vi "main.vi"() -> ()   [LabVIEW 2011]
uses:
  Sliding Menu/Sliding Menu Library/Sliding Menu xControl/Sliding Menu XControl.xctl
  Framework SubVIs/Main Type Definitions/User Interface Type Definitions.ctl
  Framework SubVIs/Main Type Definitions/UI Picture Containers.ctl
  Framework SubVIs/User Interface/UI Control Definitions/UI Configuration Information.ctl
  Framework SubVIs/Plugin Handler/Plugin Command Manager/Plugin Initialize/Plugin Handler Initialize.lvclass
  Framework SubVIs/Plugin Handler/Plugin Command Manager/Plugin Handler Command.lvclass
  Framework SubVIs/User Interface/UI Command Manager/UI Command Manager.lvclass
  Framework SubVIs/User Interface/UI Command Manager/UI Initialize/UI Initialize.lvclass
  Framework SubVIs/Plugin Handler/Plugin Command Manager/Plugin Handler Stop/Plugin Handler Stop.lvclass
  Framework SubVIs/User Interface/UI Command Manager/UI Command Manager Stop/UI Command Manager Stop.lvclass
  Framework SubVIs/User Interface/UI Command Manager/UI Resize Menu/Resize Menu.lvclass
  Framework SubVIs/Plugin Handler/Plugin Command Manager/Plugin Display UI/Plugin Display UI.lvclass
  Framework SubVIs/User Interface/UI Command Manager/UI Toggle Menu/UI Toggle Menu.lvclass
  Framework SubVIs/Plugin Handler/Plugin Command Manager/Plugin Launch Next/Plugin Load Next.lvclass
panel:
  out "Time":string
  in  "Name":string
  out "Header Image":picture
  in  "Tab Control":enum32{"Page 1", "Page 2"}(tab)
  out "Sliding Menu XControl":i32(xcontrol)
  in  "Go Home":bool
  in  "Lock Interface":bool caption="Boolean 2"
  in  "Menu":bool
  out "Footer Image":picture
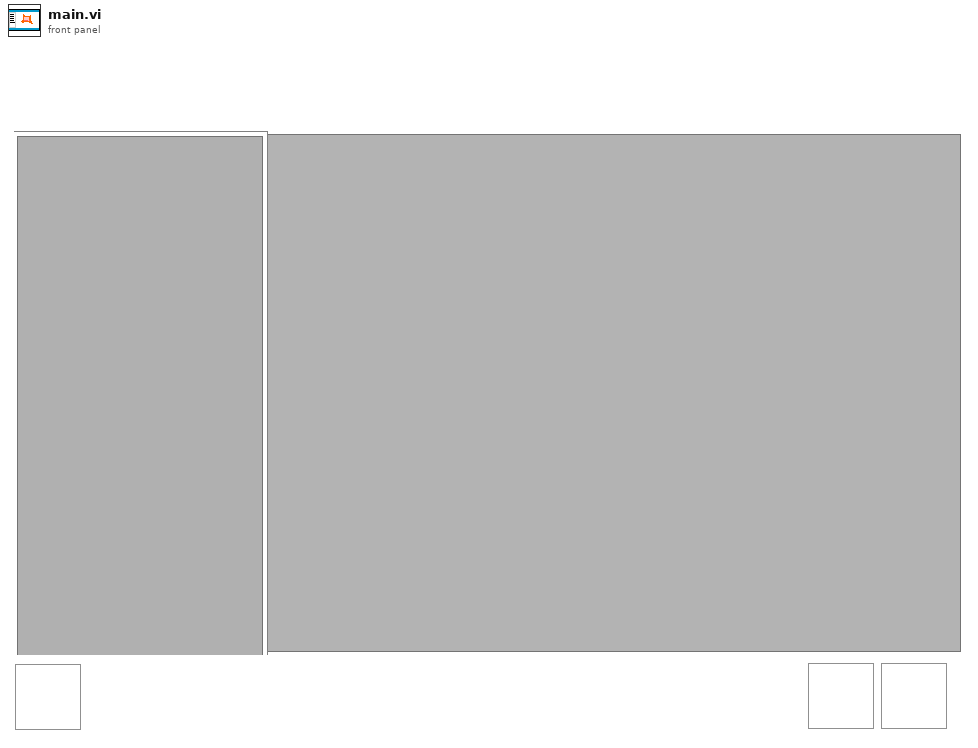
[diagram p1: front panel]
types:
  T1 = typedef "User Interface Type Definitions.ctl" = cluster{"This VI":refnum<vi>, "User Interace Plugin":refnum<vi>, "UI Picture Container References":T2, "Sliding Menu XControl":refnum<vi>, "Menu Container":refnum<vi>, "UI Configuration Information":T3, "Header Text":refnum<vi>}
  T2 = typedef "UI Picture Containers.ctl" = cluster{"Header Image":refnum<vi>, "Footer Image":refnum<vi>}
  T3 = typedef "UI Configuration Information.ctl" = cluster{"Space Between Buttons":i32, "Number of Buttons to Show":i32, "Header Image":path, "Footer Image":path}
  T4 = cluster{"Header Image":refnum<vi>, "Footer Image":refnum<vi>}
  T5 = typedef "Framework Configuration Data.ctl" = cluster{"Plugin Configuration Information":T6, "UI Configuration Information":T3}
  T6 = typedef "Plugin Configuration Information.ctl" = cluster{"Plugin Locaiton on Disk":path}
  T7 = typedef "Plugin Handler Shifter Data Definition.ctl" = cluster{"Array of Plugins":refnum<class "Generic Plugin.lvclass">[], "Plugin Configuration Information":T6, "UI Queue":refnum<queue>, "Shutdown Event":refnum<user-event>, "Menu Open Event":refnum<user-event>, "Menu Closed Event":refnum<user-event>, "Index of Plugin Showing":i32}
  T8 = enum32{"invalid app kind", "Development System", "Run Time System", "Student Edition", "Embedded LabVIEW", "Evaluation", "Custom"}
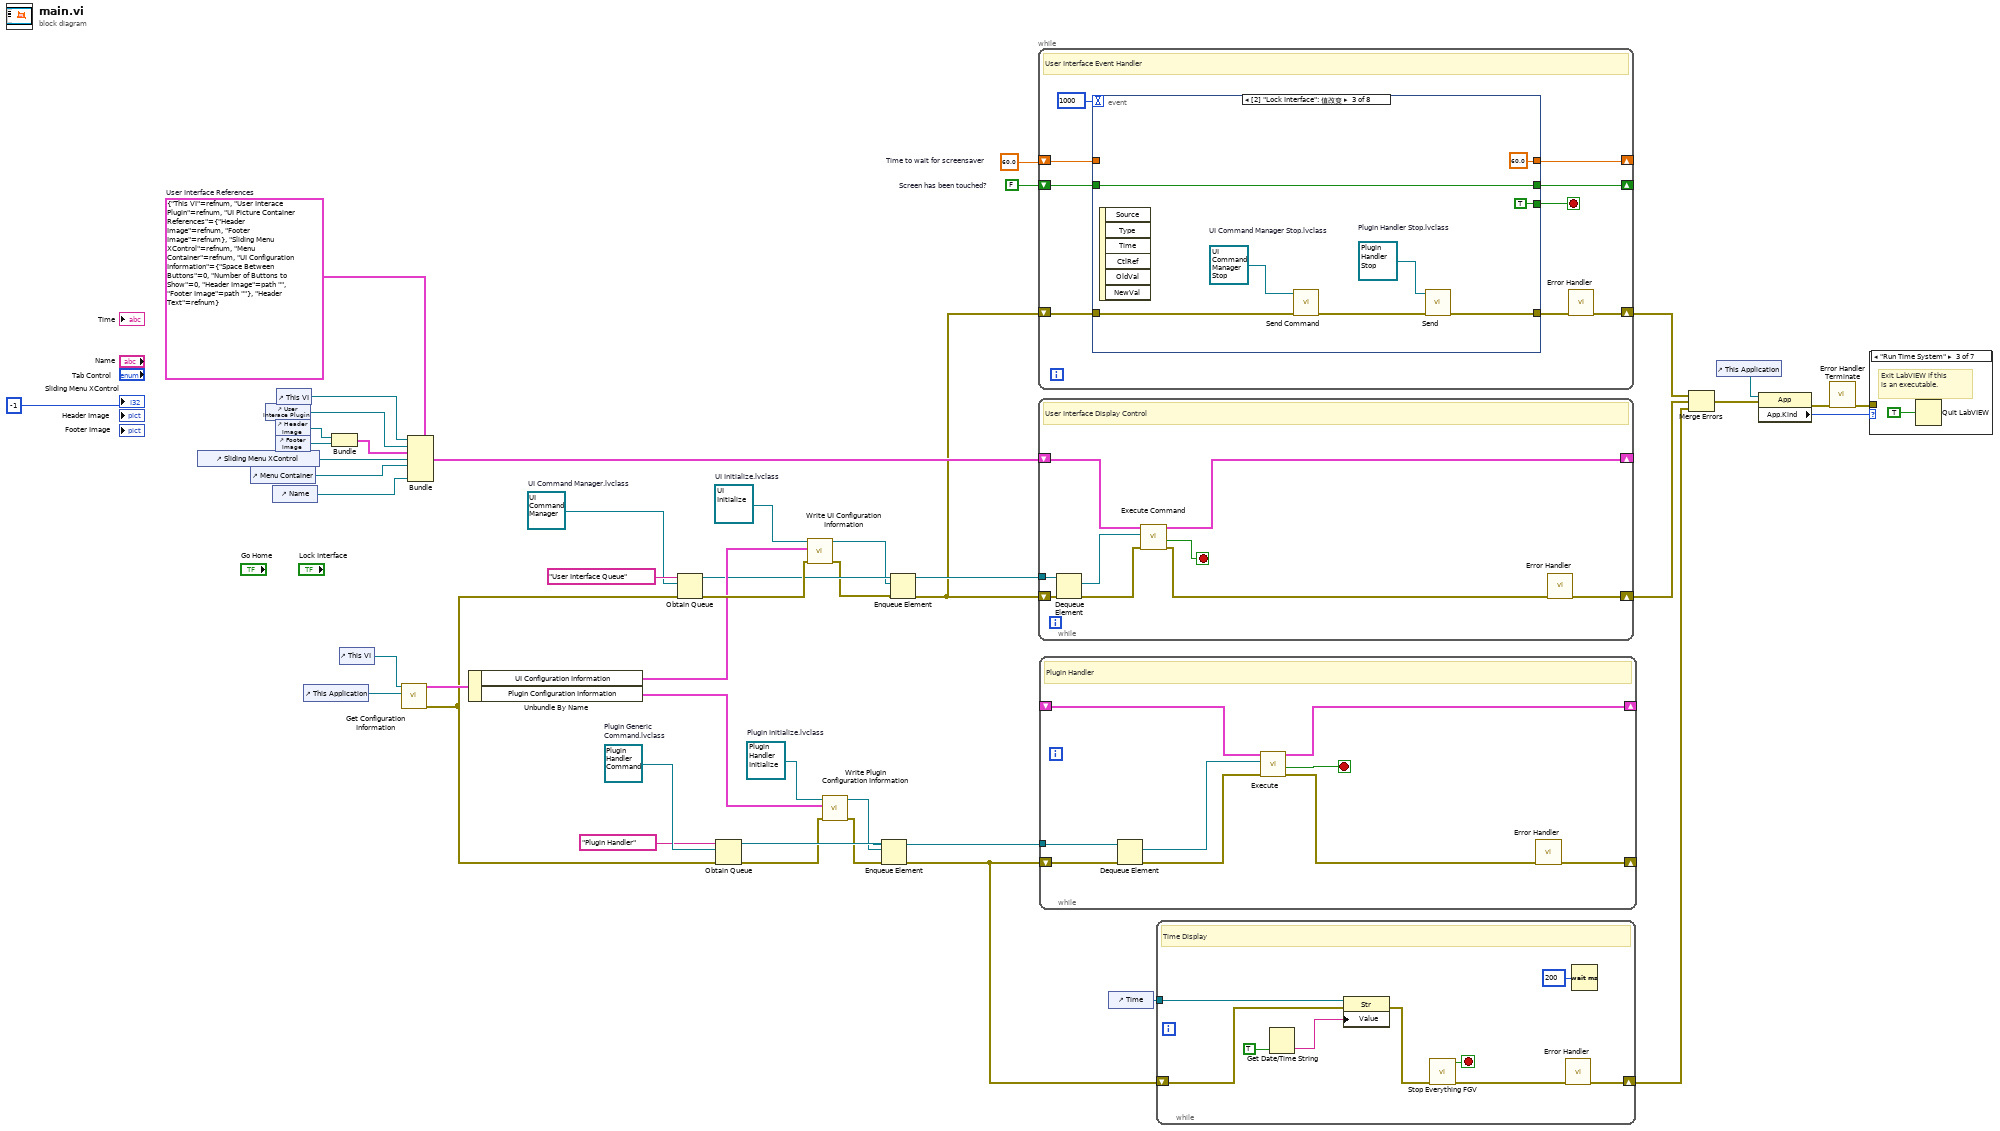
[diagram p0: block diagram]
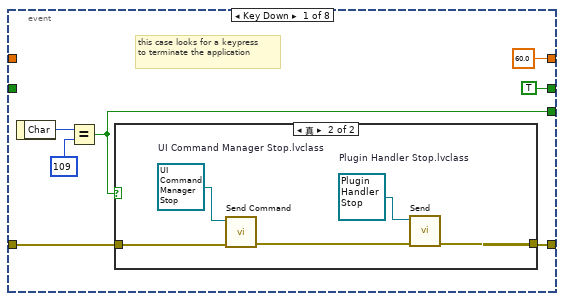
[diagram p8: hidden frame]
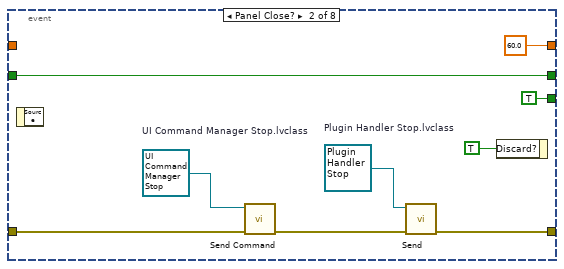
[diagram p10: hidden frame]
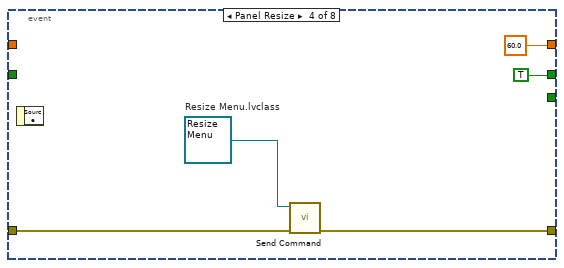
[diagram p11: hidden frame]
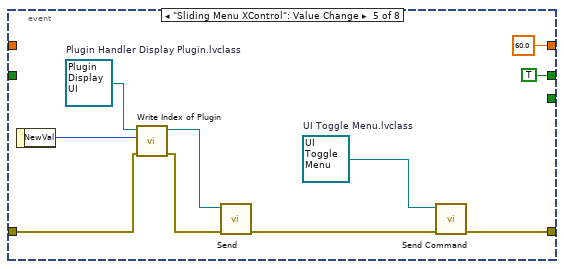
[diagram p12: hidden frame]
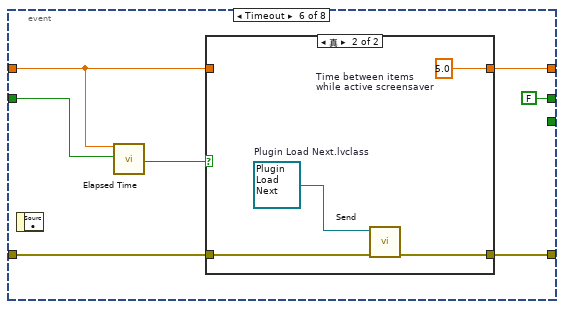
[diagram p13: hidden frame]
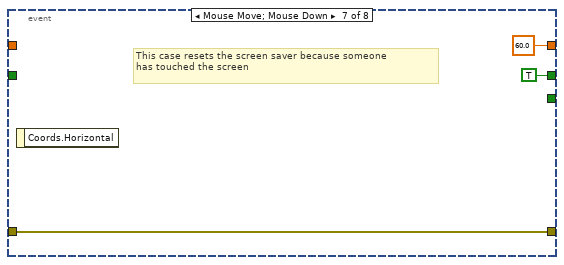
[diagram p15: hidden frame]
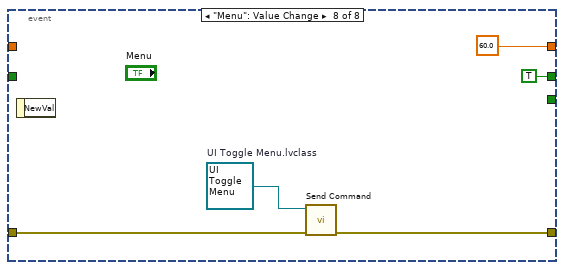
[diagram p16: hidden frame]
diagram:
  w4 = 60.0  # Time to wait for screensaver
  w6 = FALSE  # Screen has been touched?
  w15 = refnum<class "UI Initialize.lvclass"> refnum  # UI Initialize.lvclass
  w20 = refnum<class "UI Command Manager.lvclass"> refnum  # UI Command Manager.lvclass
  w24 = refnum<class "Plugin Handler Command.lvclass"> refnum  # Plugin Generic Command.lvclass
  w19 = refnum<class "Plugin Handler Initialize.lvclass"> refnum  # Plugin Initialize.lvclass
  w31 = T1 {"This VI"=refnum, "User Interace Plugin"=refnum, "UI Picture Container References"={"Header Image"=refnum, "Footer Image"=refnum}, "Sliding Menu XControl"=refnum, "Menu Container"=refnum, "UI Configuration Information"={"Space Between Buttons"=0, "Number of Buttons to Show"=0, "Header Image"=path "", "Footer Image"=path ""}, "Header Text"=refnum}  # User Interface References
  n1 = control-ref of="Sliding Menu XControl"() -> (w30:refnum<vi>)
  n2 = control-ref of="Menu Container"() -> (w32:refnum<vi>)
  n3 = control-ref of="User Interace Plugin"() -> (w25:refnum<vi>)
  n4 = control-ref of="Name"() -> (w5:refnum<vi>)
  n5 = control-ref of="Header Image"() -> (w28:refnum<vi>)
  n6 = control-ref of="Footer Image"() -> (w27:refnum<vi>)
  n7 = control-ref of="This VI"() -> (w26:refnum<vi>)
  n8 = control-ref of="This Application"() -> (w35:refnum<vi>)
  n9 = Bundle("Header Image"=w28, "Footer Image"=w27) -> (w29:T4)  [unwired: 1 in]
  n10 = control-ref of="This VI"() -> (w34:refnum<vi>)
  n11 = call "Get Configuration Information.vi"("This Application"=w35, "This VI"=w34) -> ("error out"=w12:errorcluster, "Configuration Data"=w33:T5)  [unwired: 8 in]
  n12 = Bundle(cluster=w31, "This VI"=w26, "User Interace Plugin"=w25, "UI Picture Container References"=w29, "Sliding Menu XControl"=w30, "Menu Container"=w32, "Header Text"=w5) -> (w36:T1)  [unwired: 1 in]
  n13 = Unbundle By Name(w33) -> ("UI Configuration Information"=w13:T3, "Plugin Configuration Information"=w37:T6)
  n14 = Obtain Queue(name (unnamed)="User Interface Queue", element data type=w20, error in (no error)=w12) -> (queue out=w11:refnum<queue>, error out=w14:errorcluster)  [unwired: 2 in, 1 out]
  n15 = Obtain Queue(name (unnamed)="Plugin Handler", element data type=w24, error in (no error)=w12) -> (queue out=w23:refnum<queue>, error out=w17:errorcluster)  [unwired: 2 in, 1 out]
  n16 = call "Write UI Configuration Information.vi"("error in (no error)"=w14, "UI Configuration Information"=w13, "UI Initialize in"=w15) -> ("error out"=w10:errorcluster, "UI Initialize out"=w9:refnum<class "UI Initialize.lvclass">)  [unwired: 7 in]
  n17 = call "Write Plugin Configuration Information.vi"("error in (no error)"=w17, "Plugin Configuration Information"=w37, "Plugin Handler Initialize in"=w19) -> ("error out"=w16:errorcluster, "Plugin Handler Initialize out"=w18:refnum<class "Plugin Handler Initialize.lvclass">)  [unwired: 7 in]
  n18 = Enqueue Element(queue=w23, element=w18, error in (no error)=w16) -> (queue out=w39:refnum<queue>, error out=w3:errorcluster)  [unwired: 1 in, 1 out]
  n19 = Enqueue Element(queue=w11, element=w9, error in (no error)=w10) -> (queue out=w8:refnum<queue>, error out=w7:errorcluster)  [unwired: 1 in, 1 out]
  n20 = while "User Interface Event Loop" {
    shift-right: [w52] -> w46
    shift-left: w7 -> [w54]
    shift-right: [w49] -> _
    shift-left: w6 -> [w50]
    shift-right: [w48] -> _
    shift-left: w4 -> [w47]
    stop <- w55 stop-if-true
    # "User Interface Event Handler"
    n21 = event shown="[2] \"Lock Interface\": 值改变" {
      selector: _ -> [_ _ _ _ _ _ _ _]
      dyn-events: _ -> [_ _ _ _ _ _ _ _]
      timeout: 1000 -> [_ _ _ _ _ _ _ _]
      tunnel: [w58 TRUE TRUE _ _ _ _ _] -> w55
      tunnel: w54 -> [w60 w76 w81 w87 w97 w102 w116 w120]
      tunnel: [w59 w73 w80 w86 w93 w101 w116 w119] -> w53
      tunnel: w50 -> [_ w72 w82 _ _ w107 _ _]
      tunnel: [TRUE ("Reset") w72 w82 TRUE ("Reset") TRUE ("Reset") FALSE ("Reset") TRUE ("Reset") TRUE ("Reset")] -> w49
      tunnel: [60.0 ("t") 60.0 ("t") 60.0 ("t") 60.0 ("t") 60.0 ("t") w104 60.0 ("t") 60.0 ("t")] -> w48
      tunnel: w47 -> [_ _ _ _ _ w103 _ _]
      event Key Down {
        # "this case looks for a keypress\nto terminate the application"
        n22 = event-data() -> ("Char"=w62:i16)  [unwired: 1 in]
        n23 = Equal?(x=w62, y=i16 109 ("Char")) -> (x = y?=w58:bool)
        n24 = case shown="真" w58 {
          tunnel: w60 -> [w63 w67]
          tunnel: [w63 w64] -> w59
          frame False {
          }
          frame True {
            w68 = refnum<class "UI Command Manager Stop.lvclass"> refnum  # UI Command Manager Stop.lvclass
            w66 = refnum<class "Plugin Handler Stop.lvclass"> refnum  # Plugin Handler Stop.lvclass
            n25 = call-dynamic "Send Command.vi"("error in (no error)"=w67, "UI Command Manager in"=w68) -> ("error out"=w65:errorcluster)  [unwired: 8 in, 1 out]
            n26 = call "Send.vi"("error in (no error)"=w65, "Plugin Generic Command in"=w66) -> ("error out"=w64:errorcluster)  [unwired: 8 in, 1 out]
          }
        }
      }
      event Panel Close? {
        w75 = refnum<class "Plugin Handler Stop.lvclass"> refnum  # Plugin Handler Stop.lvclass
        w77 = refnum<class "UI Command Manager Stop.lvclass"> refnum  # UI Command Manager Stop.lvclass
        n27 = event-data() -> ()  [unwired: 1 in, 1 out]
        n28 = call-dynamic "Send Command.vi"("error in (no error)"=w76, "UI Command Manager in"=w77) -> ("error out"=w74:errorcluster)  [unwired: 8 in, 1 out]
        n29 = call "Send.vi"("error in (no error)"=w74, "Plugin Generic Command in"=w75) -> ("error out"=w73:errorcluster)  [unwired: 8 in, 1 out]
        n30 = event-data("Discard?"=TRUE) -> ()  [unwired: 1 in, 1 out]
      }
      event "Lock Interface": Value Change {
        w84 = refnum<class "Plugin Handler Stop.lvclass"> refnum  # Plugin Handler Stop.lvclass
        w85 = refnum<class "UI Command Manager Stop.lvclass"> refnum  # UI Command Manager Stop.lvclass
        n31 = event-data() -> ()  [unwired: 1 in, 6 out]
        n32 = call-dynamic "Send Command.vi"("error in (no error)"=w81, "UI Command Manager in"=w85) -> ("error out"=w83:errorcluster)  [unwired: 8 in, 1 out]
        n33 = call "Send.vi"("error in (no error)"=w83, "Plugin Generic Command in"=w84) -> ("error out"=w80:errorcluster)  [unwired: 8 in, 1 out]
      }
      event Panel Resize {
        w88 = refnum<class "Resize Menu.lvclass"> refnum  # Resize Menu.lvclass
        n34 = event-data() -> ()  [unwired: 1 in, 1 out]
        n35 = call-dynamic "Send Command.vi"("error in (no error)"=w87, "UI Command Manager in"=w88) -> ("error out"=w86:errorcluster)  [unwired: 8 in, 1 out]
      }
      event "Sliding Menu XControl": Value Change {
        w95 = refnum<class "UI Toggle Menu.lvclass"> refnum  # UI Toggle Menu.lvclass
        w100 = refnum<class "Plugin Display UI.lvclass"> refnum  # Plugin Handler Display Plugin.lvclass
        n36 = event-data() -> ("NewVal"=w99:i32)  [unwired: 1 in]
        n37 = call "Write Index of Plugin.vi"("error in (no error)"=w97, "Index of Plugin"=w99, "Plugin Display UI in"=w100) -> ("error out"=w96:errorcluster, "Plugin Display UI out"=w98:refnum<class "Plugin Display UI.lvclass">)  [unwired: 7 in]
        n38 = call "Send.vi"("error in (no error)"=w96, "Plugin Generic Command in"=w98) -> ("error out"=w94:errorcluster)  [unwired: 8 in, 1 out]
        n39 = call-dynamic "Send Command.vi"("error in (no error)"=w94, "UI Command Manager in"=w95) -> ("error out"=w93:errorcluster)  [unwired: 8 in, 1 out]
      }
      event Timeout {
        n40 = event-data() -> ()  [unwired: 1 in, 1 out]
        n41 = call "Elapsed Time"("Time Target (s)"=w103, "Reset"=w107) -> ("Time has Elapsed"=w105:bool)  [unwired: 10 in, 7 out]
        n42 = case shown="真" w105 {
          tunnel: [w109 w112] -> w104
          tunnel: w103 -> [w109 _]
          tunnel: w102 -> [w108 w111]
          tunnel: [w108 w110] -> w101
          frame False {
          }
          frame True {
            w112 = 5.0  # Time between items while active screensaver
            w113 = refnum<class "Plugin Load Next.lvclass"> refnum  # Plugin Load Next.lvclass
            n43 = call "Send.vi"("error in (no error)"=w111, "Plugin Generic Command in"=w113) -> ("error out"=w110:errorcluster)  [unwired: 8 in, 1 out]
          }
        }
      }
      event Mouse Move; Mouse Down {
        # "This case resets the screen saver because someone\nhas touched the screen"
        n44 = event-data() -> ()  [unwired: 1 in, 1 out]
      }
      event "Menu": Value Change {
        w121 = refnum<class "UI Toggle Menu.lvclass"> refnum  # UI Toggle Menu.lvclass
        n45 = event-data() -> ()  [unwired: 1 in, 1 out]
        n46 = call-dynamic "Send Command.vi"("error in (no error)"=w120, "UI Command Manager in"=w121) -> ("error out"=w119:errorcluster)  [unwired: 8 in, 1 out]
      }
    }
    n47 = call "Error Handler.vi"("error in (no error)"=w53) -> ("error out"=w52:errorcluster)  [unwired: 10 in]
  }
  n48 = while {
    shift-right: [w129] -> w45
    shift-left: w7 -> [w130]
    tunnel: w8 -> [w128]
    shift-right: [w122] -> _
    shift-left: w36 -> [w127]
    stop <- w123 stop-if-true
    # "User Interface Display Control"
    n49 = Dequeue Element(queue=w128, error in (no error)=w130) -> (element=w126:refnum<class "UI Command Manager.lvclass">, error out=w125:errorcluster)  [unwired: 1 in, 2 out]
    n50 = call-dynamic "Execute Command.vi"("error in (no error)"=w125, "UI Command Manager in"=w126, "User Interface References"=w127) -> ("error out"=w124:errorcluster, "Stop?"=w123:bool, "User Interface References Out"=w122:T1)  [unwired: 5 in, 1 out]
    n51 = call "Error Handler.vi"("error in (no error)"=w124) -> ("error out"=w129:errorcluster)  [unwired: 10 in]
  }
  n52 = while {
    tunnel: w39 -> [w139]
    shift-right: [w131] -> _
    shift-left: w3 -> [w138]
    shift-right: [w136] -> _
    shift-left: _ -> [w137]
    stop <- w133 stop-if-true
    # "Plugin Handler"
    n53 = Dequeue Element(queue=w139, error in (no error)=w138) -> (element=w135:refnum<class "Plugin Handler Command.lvclass">, error out=w134:errorcluster)  [unwired: 1 in, 2 out]
    n54 = call-dynamic "Execute.vi"("error in (no error)"=w134, "Plugin Generic Command in"=w135, "Plugin Handler Shifter Data Definition"=w137) -> ("error out"=w132:errorcluster, "Stop?"=w133:bool, "Plugin Handler Shifter Data Out"=w136:T7)  [unwired: 5 in, 1 out]
    n55 = call "Error Handler.vi"("error in (no error)"=w132) -> ("error out"=w131:errorcluster)  [unwired: 10 in]
  }
  n56 = control-ref of="Time"() -> (w40:refnum<vi>)
  n57 = while {
    shift-right: [w144] -> w41
    shift-left: w3 -> [w143]
    tunnel: w40 -> [w141]
    stop <- w147 stop-if-true
    # "Time Display"
    n58 = Get Date/Time String(want seconds? (F)=TRUE) -> (time string=w140:string)  [unwired: 2 in, 1 out]
    n59 = property on="Property Node" class="Str"(reference=w141, error in=w143, "Value"=w140) -> (error out=w142:errorcluster)  [unwired: 1 out]
    n60 = call "Stop Everything FGV.vi"("error in (no error)"=w142) -> ("error out"=w145:errorcluster, "Stop?"=w147:bool)  [unwired: 9 in]
    n61 = call "Error Handler.vi"("error in (no error)"=w145) -> ("error out"=w144:errorcluster)  [unwired: 10 in]
    n62 = Wait (ms)(milliseconds to wait=u32 200) -> ()  [unwired: 1 out]
  }
  n63 = Merge Errors(w46, w45, w41) -> (w42:errorcluster)
  n64 = control-ref of="This Application"() -> (w44:refnum<vi>)
  n65 = property on="Property Node" class="App"(reference=w44, error in=w42) -> (error out=w2:errorcluster, "App.Kind"=w43:T8)  [unwired: 1 out]
  n66 = call "Error Handler Terminate.vi"("error in (no error)"=w2) -> ("error out"=w1:errorcluster)  [unwired: 10 in]
  n67 = case shown="\"Run Time System\"" w43 {
    tunnel: w1 -> [_ _ _ _ _ _ _]
    frame "invalid app kind", Default {
    }
    frame "Development System" {
    }
    frame "Run Time System" {
      # "Exit LabVIEW if this\nis an executable."
      n68 = Quit LabVIEW(quit? (T)=TRUE) -> ()
    }
    frame "Student Edition" {
    }
    frame "Embedded LabVIEW" {
    }
    frame "Evaluation" {
    }
    frame "Custom" {
    }
  }
  "Sliding Menu XControl" <- -1 ("Sliding Menu XControl")
